vi "RenameResponses.vi"(8 "error in (no error)":errorcluster, 10 "Responses":T1[](array[typedef]), 11 "BaseReader in":refnum<class "BaseReader.lvclass">) -> (0 "error out":errorcluster, 2 "Responses out":T1[](array[typedef]), 3 "BaseReader out":refnum<class "BaseReader.lvclass">)   [LabVIEW 2013, in "BaseReader.lvclass"]
doc: "Sets the name of this reader to all responses. Will leave the name of all responses untouched if this reader is not named"
uses:
  BaseReader.lvclass
  response.ctl
  driver_status.ctl
  BaseReader.lvclass/BaseReader.ctl
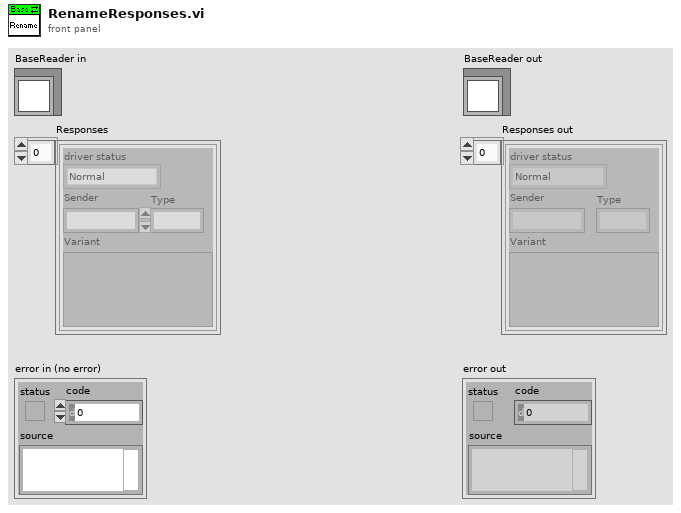
[diagram p1: front panel]
types:
  T1 = typedef "response.ctl" = cluster{"driver status":T2, "Sender":string, "Type":i32, "Variant":variant}
  T2 = typedef "driver_status.ctl" = enum16{"Normal", "Startup", "Connection lost", "Reconnected", "Timeout", "Idle", "Busy"}
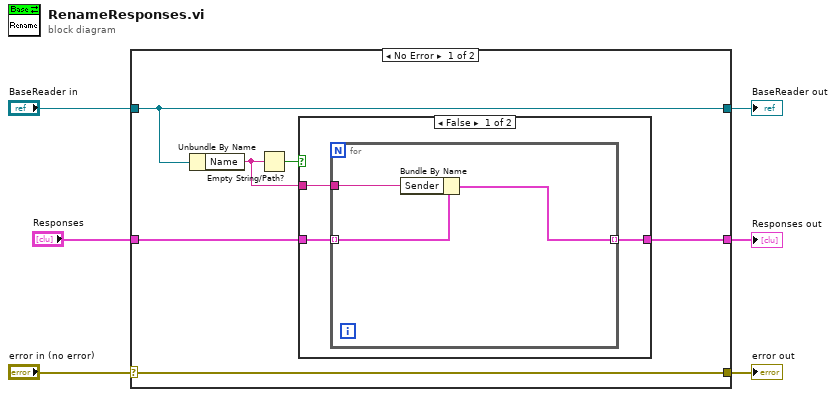
[diagram p0: block diagram]
diagram:
  n1 = case shown="No Error" "error in (no error)" {
    selector: "error in (no error)" -> [w12 w22]
    tunnel: [w12 w22] -> w5
    tunnel: [w10 w21] -> w3
    tunnel: "BaseReader in" -> [w10 w21]
    tunnel: "Responses" -> [w11 w20]
    tunnel: [w7 w20] -> w1
    frame No Error {
      n2 = Unbundle By Name(w10) -> ("Name"=w8:string)
      n3 = Empty String/Path?(string/path=w8) -> (empty?=w9:bool)
      n4 = case shown="False" w9 {
        tunnel: w11 -> [w15 w19]
        tunnel: w8 -> [w14 _]
        tunnel: [w13 w19] -> w7
        frame False {
          n5 = for {
            tunnel: w15 -> [w18] mode=indexing
            tunnel: w14 -> [w17]
            tunnel: [w16] -> w13 mode=indexing
            n6 = Bundle By Name(cluster=w18, "Sender"=w17) -> (w16:T1)
          }
        }
        frame True {
        }
      }
    }
    frame Error {
    }
  }
  "error out" <- w5
  "BaseReader out" <- w3
  "Responses out" <- w1
